vi "Mean and SD.vi"(11 "JSON Statistics in":refnum<class "JSON Statistics.lvclass">) -> (1 "SD":refnum<class "JSON Scalar.lvclass">, 2 "Is SD":bool, 3 "JSON Value":refnum<class "JSON Value.lvclass">)   [LabVIEW 2020, in "Library Commun.lvlib" / "JSON Statistics.lvclass"]
uses:
  JSON Statistics.lvclass
  JSON Value/JSON Value.lvclass
  JSON Scalar/JSON Scalar.lvclass
  C:/Users/ngarcin/OneDrive - Altyor/Standard TB/Class/JSON API/JSON Value/JSON Value.lvclass
  JSON Statistics.lvclass/JSON Statistics.ctl
  JSON Scalar/Infinity&NaN.ctl
  <vilib>/Analysis/NI_AALBase.lvlib
  support/JSON support.lvlib
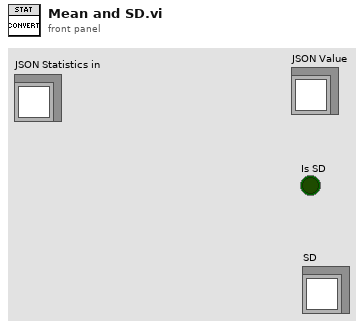
[diagram p1: front panel]
types:
  T1 = typedef "Library Commun.lvlib/JSON support.lvlib/Infinity&NaN.ctl" = enum16{"Default (null)", "Extended", "LabVIEW extensions"}
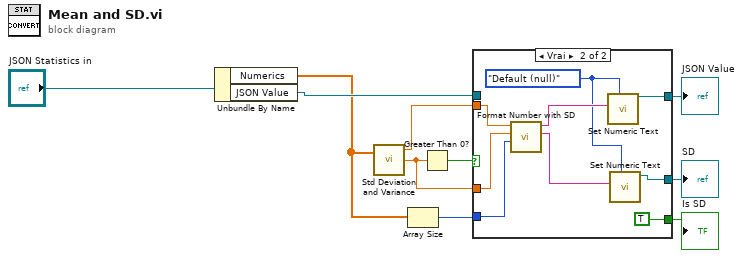
[diagram p0: block diagram]
diagram:
  n1 = Unbundle By Name("JSON Statistics in") -> ("Numerics"=w2:sgl[], "JSON Value"=w8:refnum<class "JSON Value.lvclass">)
  n2 = call <vilib>:"Std Deviation and Variance.vi"("X"=w2) -> ("mean"=w6:dbl, "standard deviation"=w5:dbl)  [unwired: 1 in, 1 out]
  n3 = Array Size(array=w2) -> (size(s)=w1:i32)
  n4 = Greater Than 0?(x=w5) -> (x > 0?=w9:bool)
  n5 = case shown="Vrai" w9 {
    tunnel: [w11 w16] -> w7
    tunnel: w8 -> [w11 _]
    tunnel: w6 -> [_ w19]
    tunnel: w5 -> [_ w18]
    tunnel: [_ TRUE] -> w4
    tunnel: [_ w14] -> w3
    tunnel: w1 -> [_ w12]
    frame False {
    }
    frame True {
      w13 = Infinity&NaN."Default (null)" ("Treatment of Infinity/NaN")
      n6 = call "Format Number with SD.vi"("Number of readings in Mean"=w12, "SD"=w18, "Mean"=w19) -> ("Formated SD"=w15:string, "Formated Mean"=w17:string)  [unwired: 7 in]
      n7 = call "Set Numeric Text.vi"("Treatment of Infinity/NaN"=w13, "Numeric Text"=w17) -> ("JSON Scalar out"=w16:refnum<class "JSON Scalar.lvclass">)  [unwired: 8 in, 1 out]
      n8 = call "Set Numeric Text.vi"("Treatment of Infinity/NaN"=w13, "Numeric Text"=w15) -> ("JSON Scalar out"=w14:refnum<class "JSON Scalar.lvclass">)  [unwired: 8 in, 1 out]
    }
  }
  "JSON Value" <- w7
  "SD" <- w3
  "Is SD" <- w4
